vi "printer.vi"() -> ()   [LabVIEW 2018]
uses:
  <vilib>/Instr/_visa.llb/VISA Configure Serial Port (Instr).vi
panel:
  in  "停止":bool
  in  "发送":bool
  in  "VISA resource name":refnum<visa-resource-name> caption="VISA资源名称"
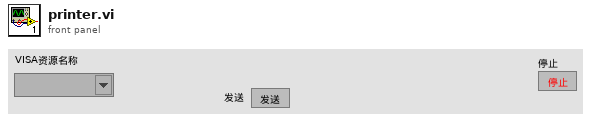
[diagram p1: front panel]
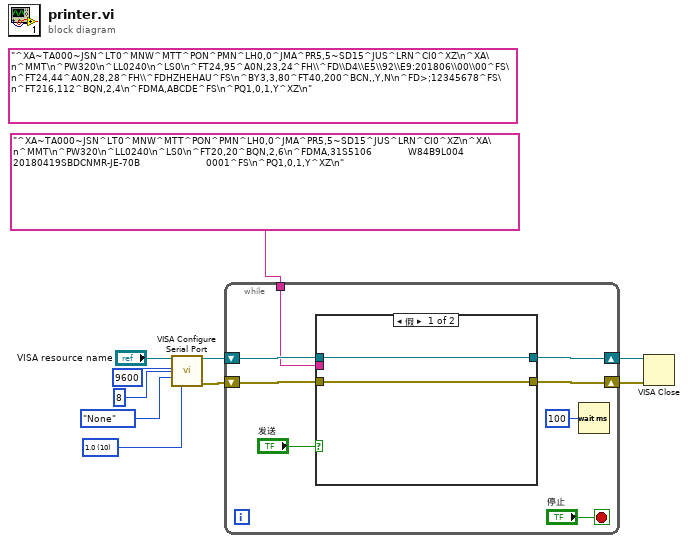
[diagram p0: block diagram]
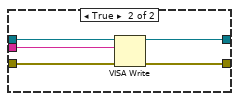
[diagram p2: hidden frame]
diagram:
  w2 = u16 10 items=["1.0"=10, "1.5"=15, "2.0"=20] ("stop bits (10: 1 bit)")
  (unwired) "^XA~TA000~JSN^LT0^MNW^MTT^PON^PMN^LH0,0^JMA^PR5,5~SD15^JUS^LRN^CI0^XZ\n^XA\n^MMT\n^PW320\n^LL0240\n^LS0\n^FT24,95^A0N,23,24^FH\\^FD\\D4\\E5\\92\\E9:201806\\00\\00^FS\n^FT24,44^A0N,28,28^FH\\^FDHZHEHAU^FS\n^BY3,3,80^FT40,200^BCN,,Y,N\n^FD>;12345678^FS\n^FT216,112^BQN,2,4\n^FDMA,ABCDE^FS\n^PQ1,0,1,Y^XZ\n" ("写入缓冲区")
  n1 = call-poly "VISA Configure Serial Port"("VISA resource name"="VISA resource name", "baud rate (9600)"=u32 9600, "data bits (8)"=u16 8, "parity (0:none)"=enum16{"None", "Odd", "Even", "Mark", "Space"}."None", "stop bits (10: 1 bit)"=w2) -> ("VISA resource name out"=w9:refnum<visa-resource-name>, "error out"=w7:errorcluster)  [unwired: 9 in]
  n2 = while {
    tunnel: "^XA~TA000~JSN^LT0^MNW^MTT^PON^PMN^LH0,0^JMA^PR5,5~SD15^JUS^LRN^CI0^XZ\n^XA\n^MMT\n^PW320\n^LL0240\n^LS0\n^FT20,20^BQN,2,6\n^FDMA,31S5106            W84B9L004        20180419SBDCNMR-JE-70B                      0001^FS\n^PQ1,0,1,Y^XZ\n" ("写入缓冲区") -> [w14]
    shift-right: [w17] -> w8
    shift-left: w9 -> [w18]
    shift-right: [w15] -> w6
    shift-left: w7 -> [w16]
    stop <- "停止" stop-if-true
    n3 = case shown="假" "发送" {
      tunnel: w18 -> [w20 w25]
      tunnel: [w20 w24] -> w17
      tunnel: w16 -> [w19 w23]
      tunnel: [w19 w22] -> w15
      tunnel: w14 -> [_ w21]
      frame False {
      }
      frame True {
        n4 = VISA Write(VISA resource name=w25, write buffer=w21, error in (no error)=w23) -> (VISA resource name out=w24:refnum<visa-resource-name>, error out=w22:errorcluster)  [unwired: 1 out]
      }
    }
    n5 = Wait (ms)(milliseconds to wait=u32 100 ("等待时间（毫秒）")) -> ()  [unwired: 1 out]
  }
  n6 = VISA Close(VISA resource name=w8, error in (no error)=w6) -> ()  [unwired: 1 out]
